vi "dvp Vi Show Property Modal Dialog.vi"(10 "hParent":u32, 11 "handle":u32) -> (3 "function return":u32(ring))   [LabVIEW 2018, in "LabViewDVPCamera.lvlib"]
doc: "LabviewDvp2Api dvpStatus dvpViShowPropertyModalDialog(dvpHandle handle, dvpUint32 hParent);"
uses:
  LabViewDVPCamera.lvlib
  LabViewDVPCamera/LabViewDVPCamera.dll
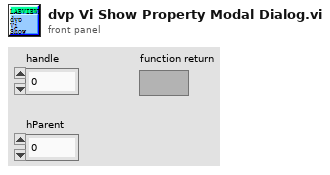
[diagram p1: front panel]
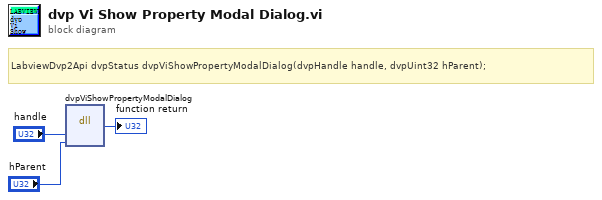
[diagram p0: block diagram]
diagram:
  # "LabviewDvp2Api dvpStatus dvpViShowPropertyModalDialog(dvpHandle handle, dvpUint32 hParent);"
  n1 = dll-call lib="C:/Program Files (x86)/DVP2 Labview cn 64/Sample/LabViewDVPCamera/LabViewDVPCamera.*" fn="dvpViShowPropertyModalDialog"("handle"="handle", "hParent"="hParent") -> (→"function return":u32)  [unwired: 5 in, 2 out]
